vi "Menu_Refnum Wire.vi"() -> (3 "Menu Items To Add":T1(array[cluster]))   [LabVIEW 2023]
uses:
  controls/action enum.ctl
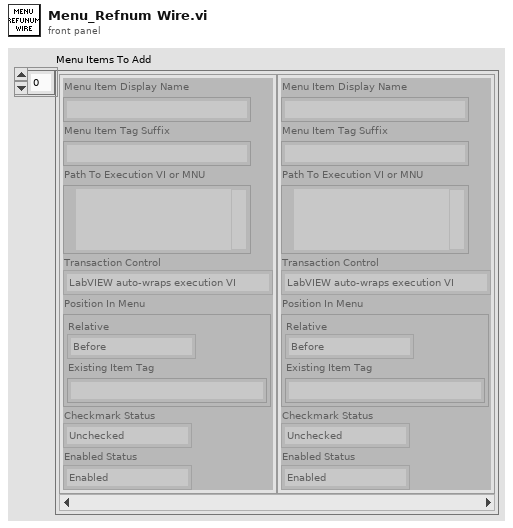
[diagram p1: front panel]
types:
  T1 = cluster{"Menu Item Display Name":string, "Menu Item Tag Suffix":string, "Path To Execution VI or MNU":path, "Transaction Control":enum8{"LabVIEW auto-wraps execution VI", "Execution VI will define if needed"}, "Position In Menu":cluster{"Relative":enum8{"Before", "Instead of", "After", "Into Submenu"}, "Existing Item Tag":string}, "Checkmark Status":enum8{"Unchecked", "Checked"}, "Enabled Status":enum8{"Enabled", "Disabled"}}[]
  T2 = typedef "action enum.ctl" = enum16{"[NONE]", "APP_SEPARATOR", "Wire Bundle", "Wire Unbundle", "Terminal Unbundle", "Terminal Bundle", "Bundler Move Up", "Bundler Move Down", "Bundler Insert", "Bundler Remove", "Bundler Remove Unwired", "Bundler Rearrange", "In Place Insert", "In Place Remove", "In Place Remove Unwired", "In Place Rearrange", "Wire Properties", "Wire Method", "Terminal Properties", "Terminal Method", "Property Move Up", "Property Move Down", "Properties Insert", "Properties Remove", "Properties Remove Unwired", "Properties Rearrange", "Method Change", "Class For Constant", "Class For Control", "Class For Node", "Class Name to Clipboard"}
  T3 = cluster{"Relative":enum8{"Before", "Instead of", "After", "Into Submenu"}, "Existing Item Tag":string}
  T4 = cluster{"Relative":enum8{"Before", "Instead of", "After", "Into Submenu"}, "Existing Item Tag":string}[]
  T5 = cluster{"Menu Item Display Name":string, "Menu Item Tag Suffix":string, "Path To Execution VI or MNU":path, "Transaction Control":enum8{"LabVIEW auto-wraps execution VI", "Execution VI will define if needed"}, "Position In Menu":cluster{"Relative":enum8{"Before", "Instead of", "After", "Into Submenu"}, "Existing Item Tag":string}, "Checkmark Status":enum8{"Unchecked", "Checked"}, "Enabled Status":enum8{"Enabled", "Disabled"}}
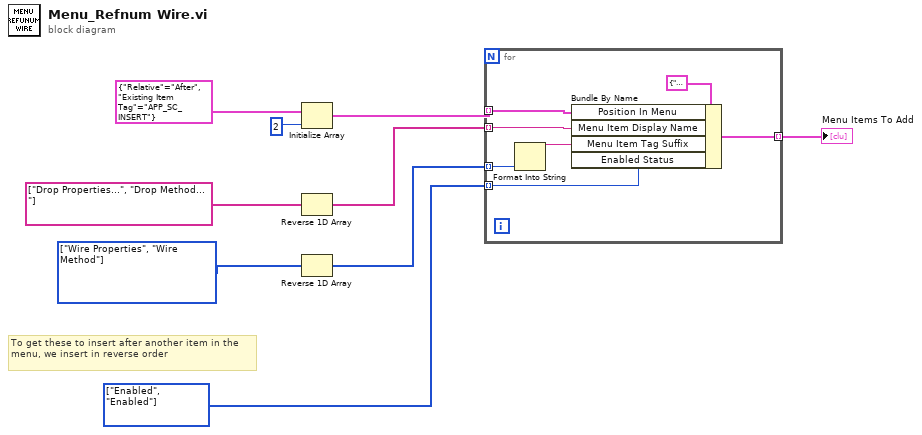
[diagram p0: block diagram]
diagram:
  w1 = T2[] [enum."Wire Properties", enum."Wire Method"] items=["[NONE]", "APP_SEPARATOR", "Wire Bundle", "Wire Unbundle", "Terminal Unbundle", "Terminal Bundle", "Bundler Move Up", "Bundler Move Down", "Bundler Insert", "Bundler Remove", "Bundler Remove Unwired", "Bundler Rearrange", "In Place Insert", "In Place Remove", "In Place Remove Unwired", "In Place Rearrange", "Wire Properties", "Wire Method", "Terminal Properties", "Terminal Method", "Property Move Up", "Property Move Down", "Properties Insert", "Properties Remove", "Properties Remove Unwired", "Properties Rearrange", "Method Change", "Class For Constant", "Class For Control", "Class For Node", "Class Name to Clipboard"] ("Array")
  w4 = enum8{"Enabled", "Disabled"}[] [enum."Enabled", enum."Enabled"] items=["Enabled", "Disabled"] ("Enabled Status")
  # "To get these to insert after another item in the menu, we insert in reverse order"
  n1 = Initialize Array(T3 {"Relative"=enum."After", "Existing Item Tag"="APP_SC_INSERT"} ("Position In Menu"), 2) -> (w3:T4)
  n2 = Reverse 1D Array(array=string[] ["Drop Properties...", "Drop Method..."]) -> (reversed array=w5:string[])
  n3 = Reverse 1D Array(array=w1) -> (reversed array=w2:T2[])
  n4 = for {
    tunnel: [w16] -> w6 mode=indexing
    tunnel: w5 -> [w15] mode=indexing
    tunnel: w3 -> [w13] mode=indexing
    tunnel: w4 -> [w12] mode=indexing
    tunnel: w2 -> [w10] mode=indexing
    n5 = Format Into String(w10) -> (resulting string=w11:string)  [unwired: 3 in, 1 out]
    n6 = Bundle By Name(cluster=T5 {"Menu Item Display Name"="", "Menu Item Tag Suffix"="", "Path To Execution VI or MNU"=path "", "Transaction Control"=enum."LabVIEW auto-wraps execution VI", "Position In Menu"={"Relative"=enum."Before", "Existing Item Tag"=""}, "Checkmark Status"=enum."Unchecked", "Enabled Status"=enum."Enabled"} ("Cluster"), "Position In Menu"=w13, "Menu Item Display Name"=w15, "Menu Item Tag Suffix"=w11, "Enabled Status"=w12) -> (w16:T5)
  }
  "Menu Items To Add" <- w6
